vi "SN_Global.vi"() -> ()   [LabVIEW 2015]
panel:
  in  "SN_Reply":refnum<queue>[](array[refnum])
  in  "SN_CmdQue":refnum<queue>[](array[refnum])
  in  "SN_ReplyRef":refnum<vi>[](array[refnum])
  # "SN_CtrlPanel"
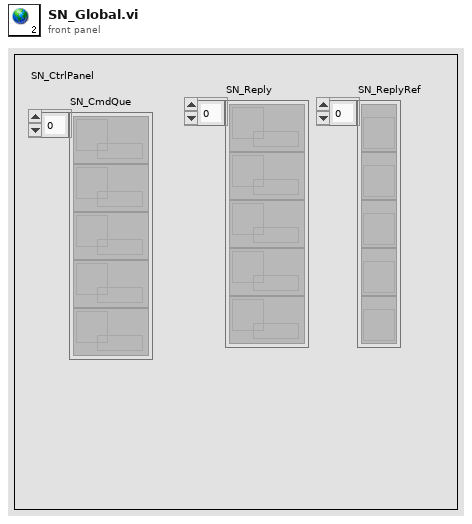
[diagram p1: front panel]
diagram:
